vi "status multifit.vi"(11 "covariance":T1) -> (2 "List Status":string[][](table), 3 "Status":i32[](array[numeric]))   [LabVIEW 2023]
uses:
  <vilib>/Analysis/Matrix/Datatypes/RealMatrix.ctl
  <vilib>/Analysis/Matrix/NI_Matrix.lvlib
panel:
  out "Error? 4":bool[](array[boolean])
  out "Error? 3":bool[][](array[boolean])
  out "Error? 2":bool[](array[boolean])
  out "Error?":bool[][](array[boolean])
  out "Upper Diagonal":dbl[][](array[numeric])
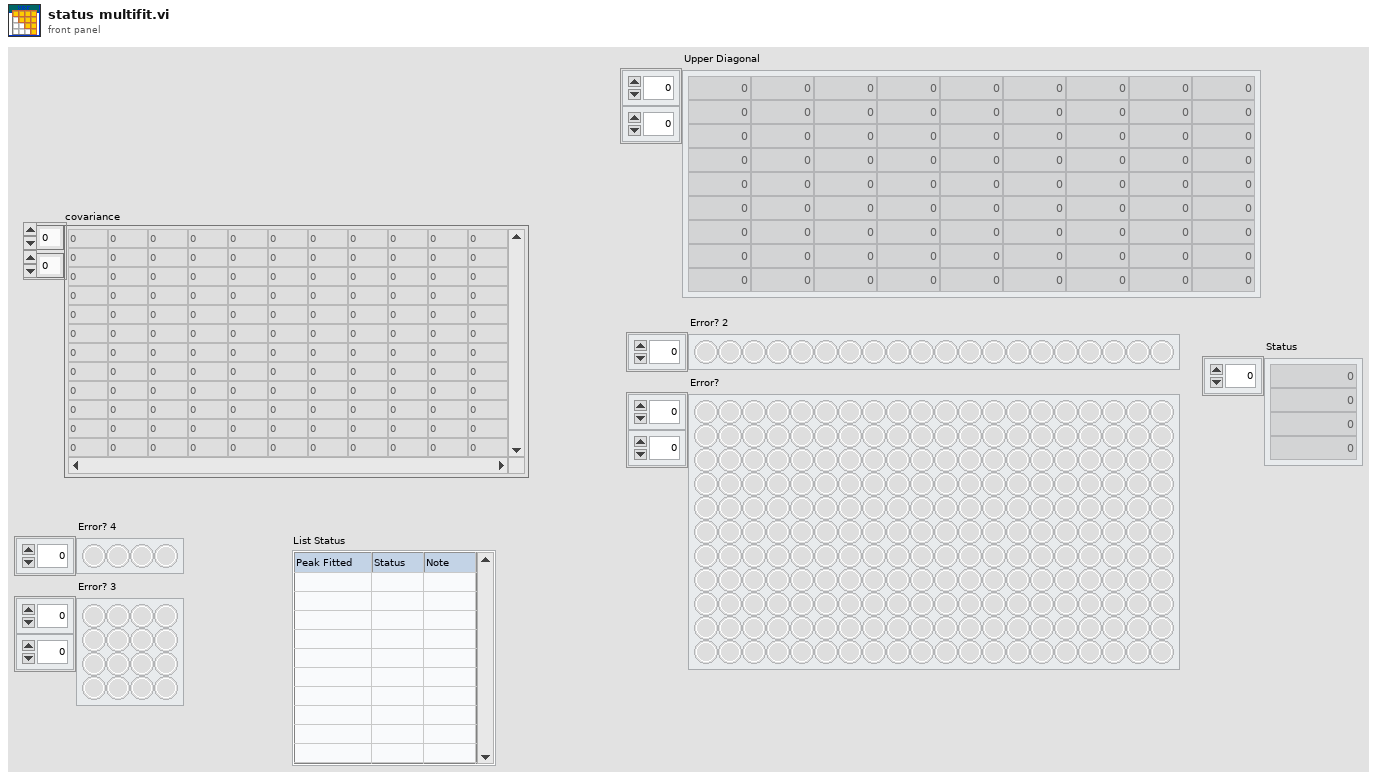
[diagram p1: front panel]
types:
  T1 = typedef "NI_Matrix.lvlib/RealMatrix.ctl" = dbl[][]
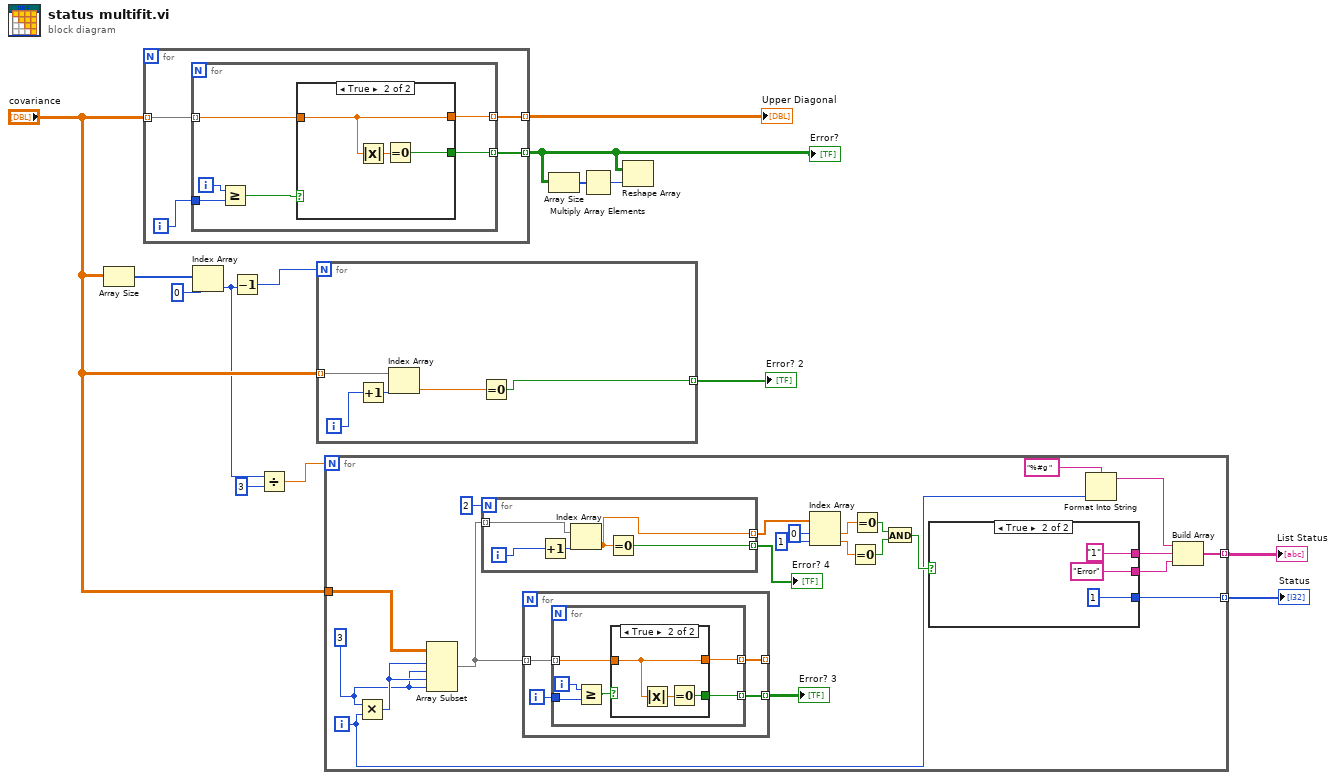
[diagram p0: block diagram]
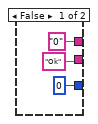
[diagram p2: hidden frame]
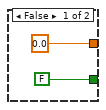
[diagram p3: hidden frame]
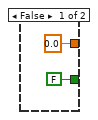
[diagram p4: hidden frame]
diagram:
  n1 = Array Size(array="covariance") -> (size(s)=w10:i32[])
  n2 = for {
    tunnel: "covariance" -> [w18] mode=indexing
    tunnel: [w16] -> w14 mode=indexing
    tunnel: [w15] -> w11 mode=indexing
    i -> [w17]
    n3 = for {
      tunnel: w18 -> [w21] mode=indexing
      tunnel: w17 -> [w23]
      tunnel: [w20] -> w16 mode=indexing
      tunnel: [w19] -> w15 mode=indexing
      i -> [w24]
      n4 = Greater Or Equal?(x=w24, y=w23) -> (x >= y?=w22:bool)
      n5 = case shown="True" w22 {
        tunnel: [0.0 ("Real Matrix Element") w28] -> w20
        tunnel: w21 -> [_ w28]
        tunnel: [FALSE w27] -> w19
        frame False {
        }
        frame True {
          n6 = Absolute Value(x=w28) -> (abs(x)=w29:dbl)
          n7 = Equal To 0?(x=w29) -> (x = 0?=w27:bool)
        }
      }
    }
  }
  "Upper Diagonal" <- w14
  "Error?" <- w11
  n8 = Index Array(array=w10, index=0) -> (element=w5:i32)
  n9 = Decrement(x=w5) -> (x-1=w8:i32)
  n10 = Divide(x=w5, y=3) -> (x/y=w4:dbl)
  n11 = for {
    N: w8 -> [_]
    tunnel: "covariance" -> [w34] mode=indexing
    tunnel: [w32] -> w7 mode=indexing
    i -> [w30]
    n12 = Increment(x=w30) -> (x+1=w31:i32)
    n13 = Index Array(array=w34, index=w31) -> (element=w33:dbl)
    n14 = Equal To 0?(x=w33) -> (x = 0?=w32:bool)
  }
  "Error? 2" <- w7
  n15 = for {
    N: w4 -> [_]
    tunnel: "covariance" -> [w54]
    tunnel: [w36] -> w2 mode=indexing
    tunnel: [w35] -> w1 mode=indexing
    i -> [w40]
    w55 = 3
    n16 = Multiply(x=w55, y=w40) -> (x*y=w56:i32)
    n17 = Array Subset(array=w54, index (row)=w56, length (row)=w55, index (col)=w56, length (col)=w55) -> (w52:T1)
    n18 = for {
      N: 2 -> [_]
      tunnel: w52 -> [w80] mode=indexing
      tunnel: [w79] -> w50 mode=indexing
      tunnel: [w78] -> w47 mode=indexing
      i -> [w81]
      n19 = Increment(x=w81) -> (x+1=w82:i32)
      n20 = Index Array(array=w80, index=w82) -> (element=w78:dbl)
      n21 = Equal To 0?(x=w78) -> (x = 0?=w79:bool)
    }
    "Error? 4" <- w50
    n22 = for {
      tunnel: w52 -> [w66] mode=indexing
      tunnel: [w64] -> _ mode=indexing
      tunnel: [w63] -> w51 mode=indexing
      i -> [w65]
      n23 = for {
        tunnel: w66 -> [w69] mode=indexing
        tunnel: w65 -> [w71]
        tunnel: [w68] -> w64 mode=indexing
        tunnel: [w67] -> w63 mode=indexing
        i -> [w72]
        n24 = Greater Or Equal?(x=w72, y=w71) -> (x >= y?=w70:bool)
        n25 = case shown="True" w70 {
          tunnel: [0.0 ("Real Matrix Element") w76] -> w68
          tunnel: w69 -> [_ w76]
          tunnel: [FALSE w75] -> w67
          frame False {
          }
          frame True {
            n26 = Absolute Value(x=w76) -> (abs(x)=w77:dbl)
            n27 = Equal To 0?(x=w77) -> (x = 0?=w75:bool)
          }
        }
      }
    }
    "Error? 3" <- w51
    n28 = Index Array(array=w47, index #1=0 ("index"), index #2=1 ("index")) -> (element #1=w45:dbl, element #2=w46:dbl)
    n29 = Equal To 0?(x=w46) -> (x = 0?=w43:bool)
    n30 = Equal To 0?(x=w45) -> (x = 0?=w44:bool)
    n31 = And(x=w44, y=w43) -> (x .and. y?=w42:bool)
    n32 = case shown="True" w42 {
      tunnel: ["0" ("input 1") "1" ("input 1")] -> w38
      tunnel: ["Ok" ("input 1") "Error" ("input 1")] -> w37
      tunnel: [0 1] -> w35
      frame False {
      }
      frame True {
      }
    }
    n33 = Format Into String(format string="%#g " ("resulting string"), w40) -> (resulting string=w39:string)  [unwired: 2 in, 1 out]
    n34 = Build Array(w39, w38, w37) -> (w36:string[])
  }
  "List Status" <- w2
  "Status" <- w1
  n35 = Array Size(array=w11) -> (size(s)=w13:i32[])
  n36 = Multiply Array Elements(1:w13) -> (0:w12:i32)
  n37 = Reshape Array(w11, w12) -> ()  [unwired: 1 out]
